vi "SubVI_1D_Cholesky_generalization_FPGA_SGL.vi"(8 "error in (no error)":errorcluster, 9 "M":dbl[][](array[numeric]), 10 "K":dbl[][](array[numeric]), 11 "Refnum in":refnum<k20>) -> (0 "error out":errorcluster, 2 "C":dbl[][](array[numeric]), 3 "Refnum out":refnum<k20>)   [LabVIEW 2019]
uses:
  <vilib>/Utility/error.llb/Error Cluster From Error Code.vi
  <vilib>/rvi/errors/niLvFpgaAdjustHostInterfaceError.vi
  <vilib>/FPGAPlugInAG/Dynamic/niLvFpga_Run_Dynamic.vi
  <vilib>/Analysis/baseanly.llb/Real Inverse Matrix.vi
  <vilib>/Analysis/Matrix/Numeric/Multiply/Multiply - RM,RM.vi
  <vilib>/Analysis/Matrix/Numeric/Add/Add - RM,RM.vi
  <vilib>/Analysis/Matrix/Numeric/Conversions/Matrix To Array - RM.vi
  <vilib>/rvi/interface/nirviMethod/nirviMethod.xnode
  <vilib>/Analysis/NI_AALBase.lvlib
  <vilib>/Analysis/Matrix/NI_Matrix.lvlib
  <vilib>/rvi/errors/niLvFpgaMergeErrorWithErrorCode.vi
  <vilib>/FPGAPlugInAG/Dynamic/niLvFpga_ReadFifo_Dynamic.vi
  <vilib>/FPGAPlugInAG/Dynamic/niLvFpga_WriteFifo_Dynamic.vi
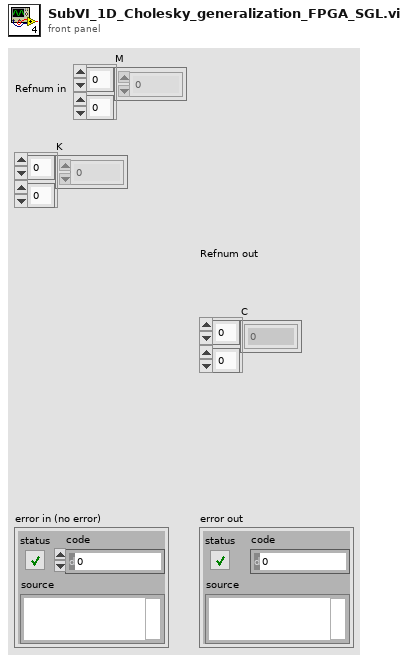
[diagram p1: front panel]
types:
  T1 = typedef "NI_Matrix.lvlib/RealMatrix.ctl" = dbl[][]
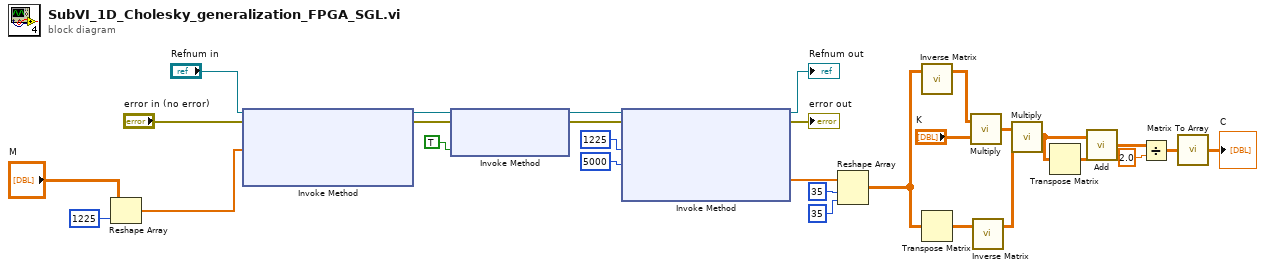
[diagram p0: block diagram]
diagram:
  n1 = Reshape Array("M", 1225 ("dimension size")) -> (w1:dbl[])
  n2 = xnode "Invoke Method"("FPGA VI Reference In"="Refnum in", "error in"="error in (no error)", "Data"=w1) -> ("FPGA VI Reference Out"=w16:refnum<k20>, "error out"=w17:errorcluster)  [unwired: 1 in, 1 out]
  n3 = xnode "Invoke Method"("FPGA VI Reference In"=w16, "error in"=w17, "Wait Until Done (F)"=TRUE) -> ("FPGA VI Reference Out"=w18:refnum<k20>, "error out"=w19:errorcluster)
  n4 = xnode "Invoke Method"("FPGA VI Reference In"=w18, "error in"=w19, "Number of Elements"=u32 1225, "Timeout (ms)"=5000) -> ("FPGA VI Reference Out"=→"Refnum out":refnum<k20>, "error out"=→"error out":errorcluster, "Data"=w23:sgl[])  [unwired: 1 out]
  n5 = Reshape Array(w23, 35 ("dimension size"), 35 ("dimension size")) -> (w24:sgl[][])
  n6 = call-poly <vilib>:"Inverse Matrix.vi"("Input Matrix"=w24) -> ("Inverse Matrix"=w7:T1)  [unwired: 1 in, 1 out]
  n7 = Transpose Matrix(1:w24) -> (0:w14:dbl[][])
  n8 = call-poly <vilib>:"Multiply.vi"("Real Matrix B"="K", "Real Matrix A"=w7) -> ("A * B"=w9:T1)
  n9 = call-poly <vilib>:"Inverse Matrix.vi"("Input Matrix"=w14) -> ("Inverse Matrix"=w8:T1)  [unwired: 1 in, 1 out]
  n10 = call-poly <vilib>:"Multiply.vi"("Real Matrix B"=w8, "Real Matrix A"=w9) -> ("A * B"=w10:T1)
  n11 = Transpose Matrix(1:w10) -> (0:w11:T1)
  n12 = call-poly <vilib>:"Add.vi"("Real Matrix B"=w11, "Real Matrix A"=w10) -> ("A + B"=w13:T1)
  n13 = Divide(x=w13, y=2.0) -> (x/y=w28:T1)
  n14 = call-poly <vilib>:"Matrix To Array.vi"("Real Matrix"=w28) -> ("Real 2D Array"=→"C":dbl[][])
